vi "Analysis.Result Summaries to First and Last Pass Result Info_V2.vi"(11 "ResultSum":T3) -> (2 "Images":T1[](array[typedef]), 3 "Pareto Gen Input":T2)   [LabVIEW 2024]
uses:
  Analysis.Result Summary_V2.ctl
  Analysis.Fail Paredo Gen Input_V2.ctl
  Analysis.DataFG.Image File List.ctl
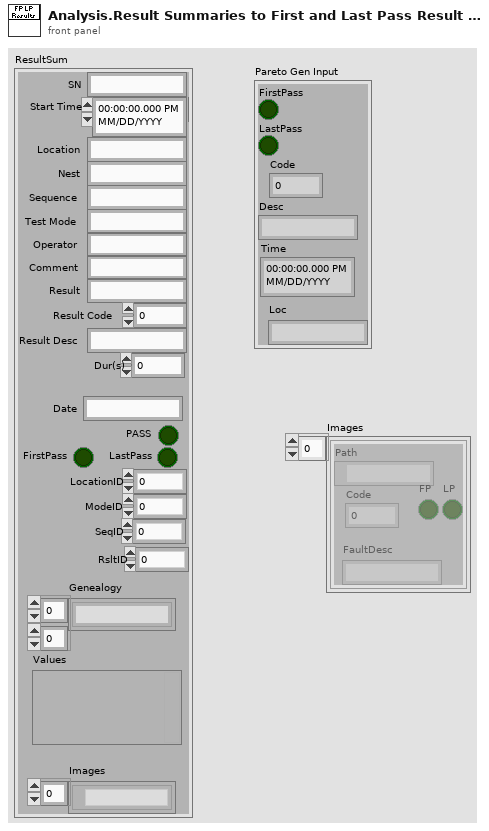
[diagram p1: front panel]
types:
  T1 = typedef "Analysis.DataFG.Image File List.ctl" = cluster{"Path":path, "Code":i32, "LP":bool, "FP":bool, "FaultDesc":string}
  T2 = typedef "Analysis.Fail Paredo Gen Input_V2.ctl" = cluster{"FirstPass":bool, "LastPass":bool, "Code":i32, "Desc":string, "Time":timestamp, "Loc":string}
  T3 = typedef "Analysis.Result Summary_V2.ctl" = cluster{"SN":string, "Start Time":timestamp, "Location":string, "Nest":string, "Sequence":string, "Operator":string, "Test Mode":string, "Comment":string, "Result":string, "Result Code":i32, "Result Desc":string, "Date":string, "Dur(s)":dbl, "PASS":bool, "FirstPass":bool, "LastPass":bool, "LocationID":i32, "ModeID":i32, "SeqID":i32, "RsltID":i32, "Genealogy":string[][], "Values":variant, "Images":path[]}
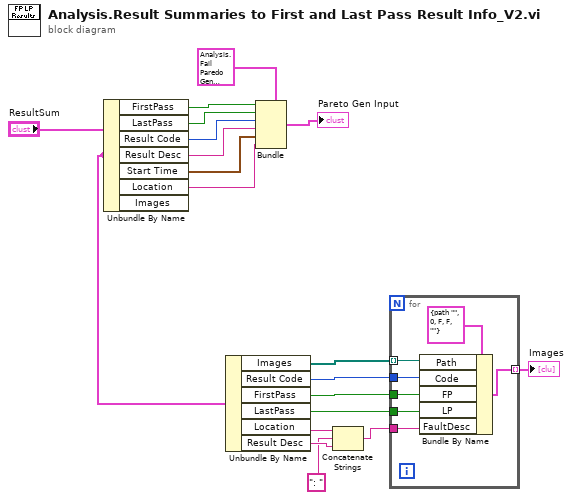
[diagram p0: block diagram]
diagram:
  n1 = Unbundle By Name("ResultSum") -> ("FirstPass"=w18:bool, "LastPass"=w17:bool, "Result Code"=w16:i32, "Result Desc"=w15:string, "Start Time"=w13:timestamp, "Location"=w11:string)  [unwired: 1 out]
  n2 = Unbundle By Name("ResultSum") -> ("Images"=w10:path[], "Result Code"=w9:i32, "FirstPass"=w8:bool, "LastPass"=w7:bool, "Location"=w4:string, "Result Desc"=w3:string)
  n3 = Bundle(cluster=T2 {"FirstPass"=FALSE, "LastPass"=FALSE, "Code"=0, "Desc"="", "Time"=timestamp(0 s since 1904-01-01), "Loc"=""} ("Pareto Gen Input"), "FirstPass"=w18, "LastPass"=w17, "Code"=w16, "Desc"=w15, "Time"=w13, "Loc"=w11) -> (→"Pareto Gen Input":T2)
  n4 = Concatenate Strings(w4, ": ", w3) -> (w2:string)
  n5 = for {
    tunnel: w10 -> [w24] mode=indexing
    tunnel: w9 -> [w23]
    tunnel: [w22] -> w5 mode=indexing
    tunnel: w8 -> [w21]
    tunnel: w7 -> [w20]
    tunnel: w2 -> [w19]
    n6 = Bundle By Name(cluster=T1 {"Path"=path "", "Code"=0, "LP"=FALSE, "FP"=FALSE, "FaultDesc"=""} ("Image File"), "Path"=w24, "Code"=w23, "FP"=w21, "LP"=w20, "FaultDesc"=w19) -> (w22:T1)
  }
  "Images" <- w5
